vi "RNN_iterate_through_sequence.vi"() -> ()   [LabVIEW 2014]
uses:
  <vilib>/Analysis/Matrix/Datatypes/RealMatrix.ctl
  <vilib>/Analysis/Matrix/NI_Matrix.lvlib
panel:
  out "Loss Array":dbl[](array[numeric]) format="%_8f"
  out "Loss (total)":dbl format="%_8f"
  in  "Number of Batches":i32
  out "h_latest":T1=[[0.9959918876590693], [-0.9609924209716473]]
  out "params_":T2={"Wxh"=[[0.578129, 2.470063497819347, -0.0219857], [-2.46959, 0.1272618664533515, 2.449614362]], "Whh"=[[-1.3996, 0.961745], [0.364566, -0.477064]], "bh"=[[0.43547749781934725], [-1.8859871335466485]], "Why"=[[-0.5586160007940589, 0.6646920008529518], [-1.8789985538066074, 0.48803595038059944], [-0.23091199894822387, -0.2339880011297829]], "by"=[[-0.4284170007877064], [-0.5403199541761617], [-0.9844818989566383]]} {"Wxh" format="%_8f"; "Whh" format="%_8f"; "bh" format="%_8f"; "Why" format="%_8f"; "by" format="%_8f"}
  in  "learning_rate":dbl=0.1
  out "dParams_":T3={"dWxh"=[[0.0, 0.0019862373697962215, 0.0], [0.0, -0.06118825535684556, 0.0]], "dWhh"=[[0.0, 0.0], [0.0, 0.0]], "dbh"=[[0.0019862373697962215], [-0.06118825535684556]], "dWhy"=[[-0.7935213511320954, 0.7656367624734651], [0.10403870131705772, -0.10038274878765777], [0.6894826498150377, -0.6652540136858074]], "dby"=[[-0.796714673045329], [0.10445737822381787], [0.6922572948215111]]} {"dWxh" format="%_8f"; "dWhh" format="%_8f"; "dbh" format="%_8f"; "dWhy" format="%_8f"; "dby" format="%_8f"}
  in  "targets":i64[](array[numeric])=[0]
  in  "_inputs":i32[](array[numeric])=[1]
  in  "_params":T2={"Wxh"=[[0.578129, 2.569937, -0.0219857], [-2.46959, 0.027262, 2.449614362]], "Whh"=[[-1.3996, 0.961745], [0.364566, -0.477064]], "bh"=[[0.535351], [-1.985987]], "Why"=[[-0.658616, 0.764692], [-1.7789986, 0.388036], [-0.130912, -0.333988]], "by"=[[-0.528417], [-0.44032], [-0.8844819]]} {"Wxh" format="%_8f"; "Whh" format="%_8f"; "bh" format="%_8f"; "Why" format="%_8f"; "by" format="%_8f"}
  in  "_hprev":T1=[[0.0], [0.0]]
  in  "_vocab size":i32=3
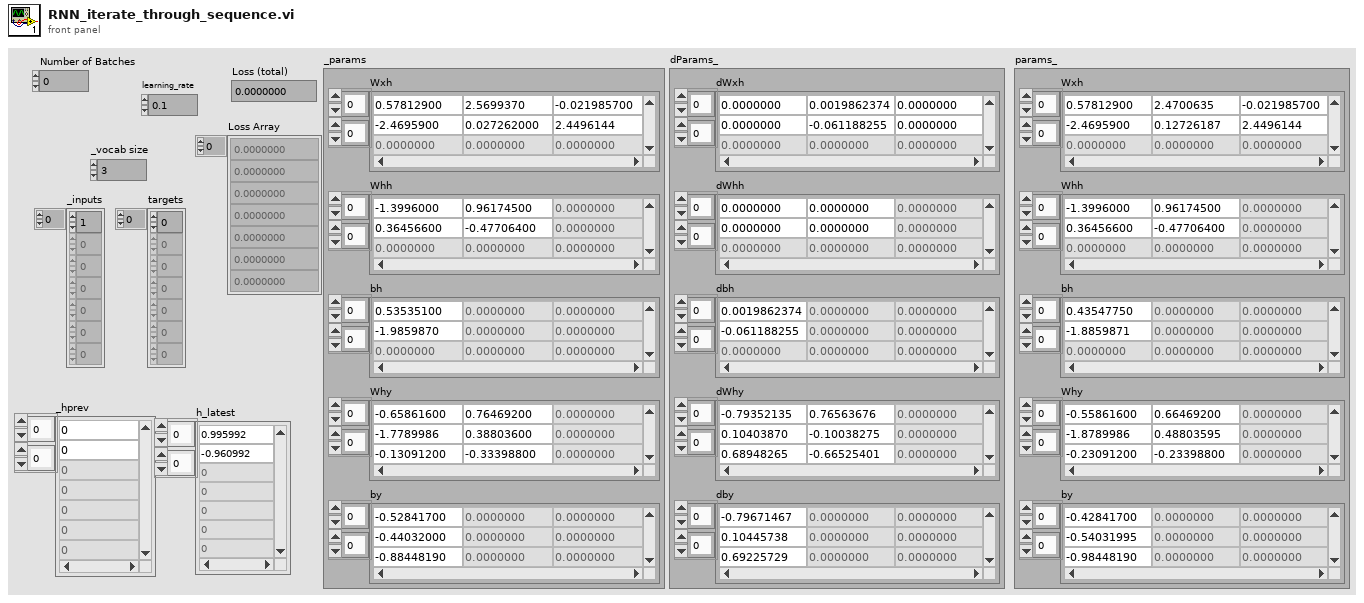
[diagram p1: front panel]
types:
  T1 = typedef "NI_Matrix.lvlib/RealMatrix.ctl" = dbl[][]
  T2 = cluster{"Wxh":T1, "Whh":T1, "bh":T1, "Why":T1, "by":T1}
  T3 = cluster{"dWxh":T1, "dWhh":T1, "dbh":T1, "dWhy":T1, "dby":T1}
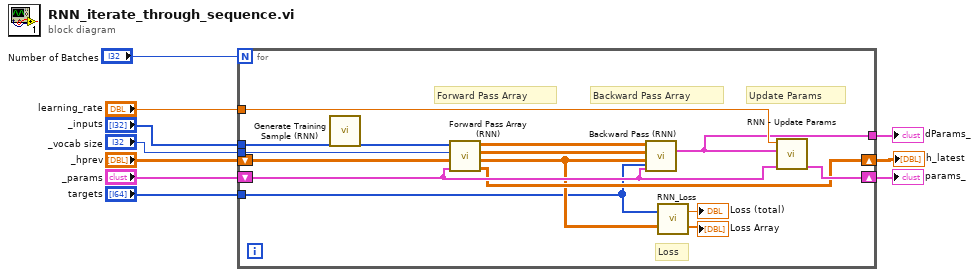
[diagram p0: block diagram]
diagram:
  n1 = for {
    N: "Number of Batches" -> [_]
    tunnel: "_inputs" -> [w22]
    tunnel: "_vocab size" -> [w20]
    tunnel: "learning_rate" -> [w19]
    tunnel: [w17] -> w5
    tunnel: "targets" -> [w13]
    shift-right: [w15] -> w3
    shift-left: "_hprev" -> [w21]
    shift-right: [w18] -> w6
    shift-left: "_params" -> [w16]
    # "Loss"
    # "Update Params"
    # "Backward Pass Array"
    # "Forward Pass Array"
    n2 = call "Generate Training Sample (RNN).vi"() -> ()  [unwired: 3 in, 2 out]
    n3 = call "Forward Pass Array (RNN).vi"("inputs"=w22, "vocab size"=w20, "hprev"=w21, "params"=w16) -> ("xs"=w23:dbl[][][], "hs"=w24:dbl[][][], "ps"=w14:dbl[][][], "h_latest"=w15:T1)  [unwired: 3 in]
    n4 = call "Backward Pass (RNN).vi"("xs"=w23, "hs"=w24, "ps"=w14, "targets"=w13, "params"=w16) -> ("dParams_"=w17:T3)  [unwired: 10 in]
    n5 = call "RNN_Loss.vi"("targets"=w13, "ps"=w14) -> ("Loss (total)"=→"Loss (total)":dbl, "Loss Array"=→"Loss Array":dbl[])  [unwired: 16 in]
    n6 = call "RNN - Update Params.vi"("learning_rate"=w19, "dParams"=w17, "_params"=w16) -> ("params_"=w18:T2)  [unwired: 5 in]
  }
  "dParams_" <- w5
  "params_" <- w6
  "h_latest" <- w3
